vi "Header.vi"() -> ()   [LabVIEW 2011]
uses:
  <vilib>/Utility/miscctls.llb/LVPointTypeDef.ctl
  Globals/Global VI.vi
  Globals/Global Recipe.vi
panel:
  out "System Status :":u16(ring) items=["NOT READY", "E-STOPPED", "FAULTED", "PAUSING...", "PAUSED", "IDLE", "RUNNING", "UNCALIBRATED", "CALIBRATING...", "POWER OFF", "POWERING ON...", "MANUAL MODE", "CONNECTING..."]
  out "Faulted":bool
  in  "Previous Button":bool
  in  "Next Button":bool
  in  "Last Button":bool
  in  "First Button":bool
  in  "Login Button":bool
  out "Date/Time":string="Date\nTime"
  out "String":string
  out "Operator":string
  out "System Info":string="System Idle"
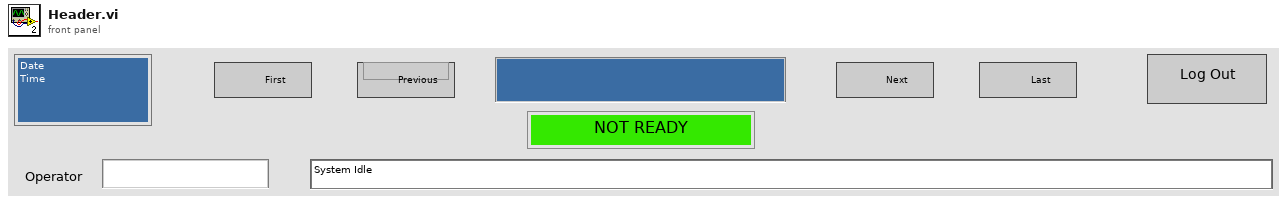
[diagram p1: front panel]
types:
  T1 = typedef "LVPointTypeDef.ctl" = cluster{"Horizontal":i16, "Vertical":i16}
  T2 = enum16{"Always On", "Always Off", "Off While Running"}
  T3 = typedef "LVRectTypeDef.ctl" = cluster{"left":i16, "top":i16, "right":i16, "bottom":i16}
  T4 = typedef "LVAllMonitorsDisplayTypeDef.ctl" = cluster{"Bounds":cluster{"Left":i16, "Top":i16, "Right":i16, "Bottom":i16}, "Depth":i16}[]
  T5 = cluster{"Bounds":cluster{"Left":i16, "Top":i16, "Right":i16, "Bottom":i16}, "Depth":i16}
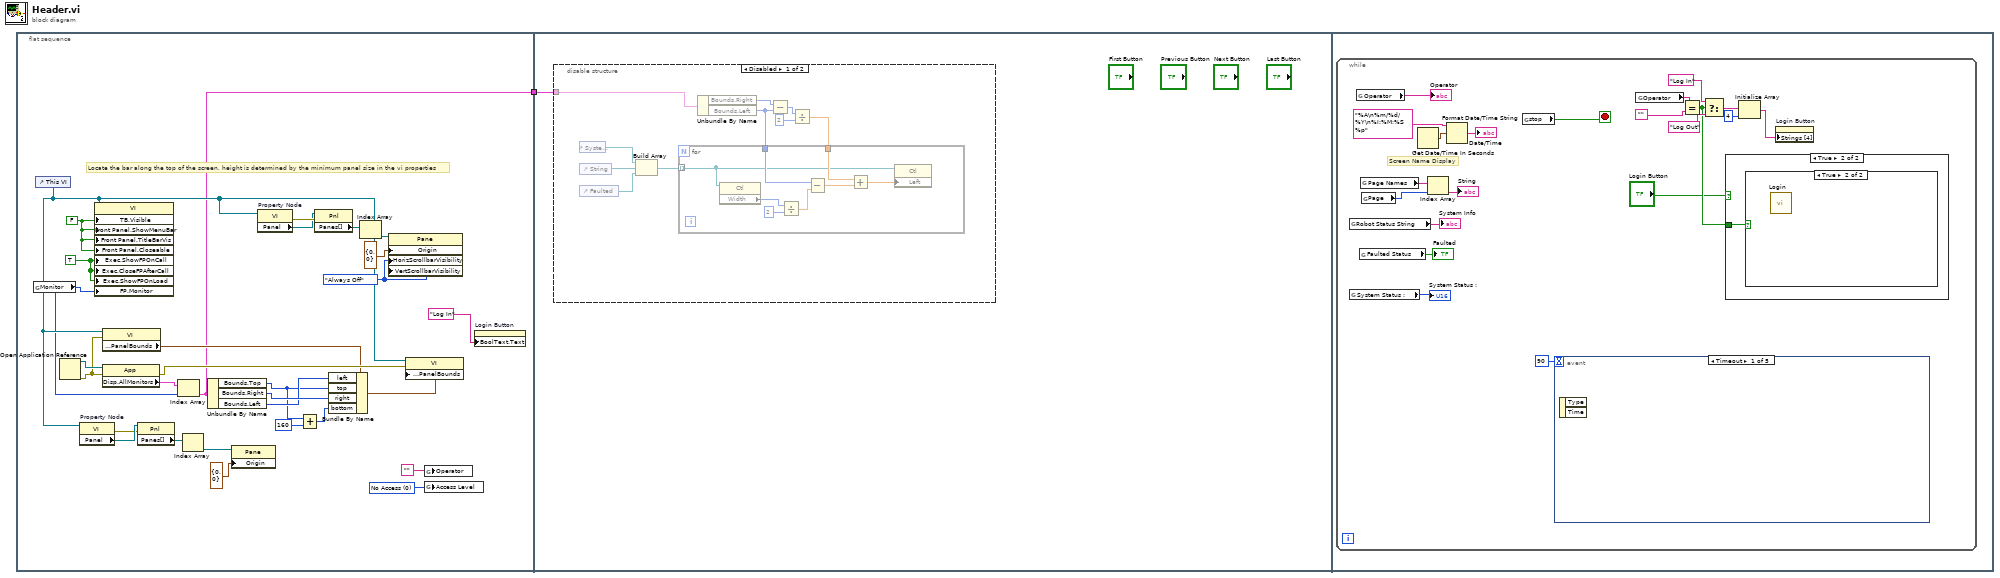
[diagram p0: block diagram]
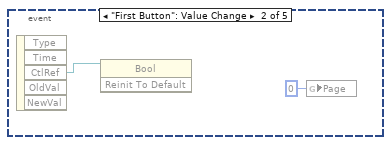
[diagram p3: hidden frame]
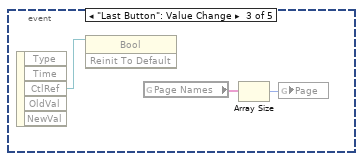
[diagram p4: hidden frame]
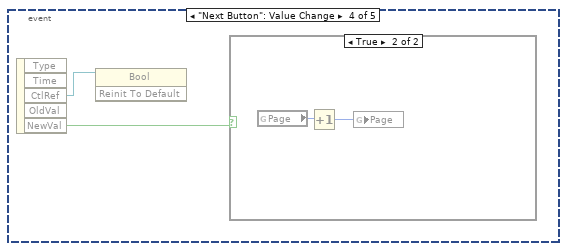
[diagram p5: hidden frame]
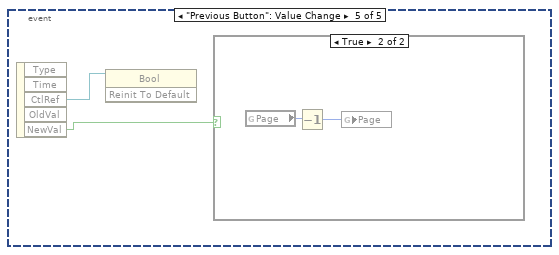
[diagram p7: hidden frame]
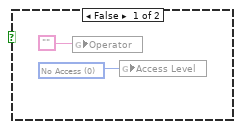
[diagram p10: hidden frame]
diagram:
  n1 = flat-sequence {
    tunnel: [w3] -> w1
    tunnel: w1 -> [w32]
    frame #0 {
      w6 = u16 0 items=["No Access", "Operator", "Engineer/Tech"] ("Access Level")
      w9 = TRUE ("Execution:Show Front Panel On Call")
      w8 = FALSE ("Tool Bar:Visible")
      w11 = T2."Always Off" ("Horizontal Scrollbar Visibility")
      # "Locate the bar along the top of the screen, height is determined by the minimum panel size in the vi properties"
      n2 = global read "Global VI.vi" "Monitor"() -> (w2:u16)
      n3 = control-ref of="This VI"() -> (w7:refnum<vi>)
      n4 = Open Application Reference() -> (0:w27:errorcluster, 3:w28:refnum<vi>)  [unwired: 4 in]
      n5 = property on="Property Node" class="VI"(reference=w7) -> (error out=w25:errorcluster, "Panel"=w26:refnum<vi>)  [unwired: 1 in, 1 out]
      n6 = property class="VI"(reference=w7, "TB.Visible"=w8, "Front Panel.ShowMenuBar"=w8, "Front Panel.TitleBarVis"=w8, "Front Panel.Closeable"=w8, "Exec.ShowFPOnCall"=w9, "Exec.CloseFPAfterCall"=w9, "Exec.ShowFPOnLoad"=w9, "FP.Monitor"=w2) -> ()  [unwired: 1 in, 2 out]
      n7 = property class="VI"(reference=w7, error in=w27) -> ("Front Panel.PanelBounds"=w21:T3)  [unwired: 2 out]
      n8 = property class="App"(reference=w28, error in=w27) -> (error out=w30:errorcluster, "Disp.AllMonitors"=w31:T4)  [unwired: 1 out]
      n9 = property class="Pnl"(reference=w26, error in=w25) -> ("Panes[]"=w24:refnum<vi>[])  [unwired: 2 out]
      n10 = Index Array(array=w31, index=w2) -> (element=w3:T5)
      n11 = Index Array "Index Array"(array=w24) -> (element=w23:refnum<vi>)  [unwired: 1 in]
      n12 = Unbundle By Name(w3) -> ("Bounds.Top"=w18:i16, "Bounds.Right"=w20:i16, "Bounds.Left"=w19:i16)
      n13 = property class="Pane"(reference=w23, "Origin"=T1 {"Horizontal"=0, "Vertical"=0}) -> ()  [unwired: 1 in, 2 out]
      n14 = property on="Property Node" class="VI"(reference=w7) -> (error out=w13:errorcluster, "Panel"=w12:refnum<vi>)  [unwired: 1 in, 1 out]
      n15 = Add(x=w18, y=i16 160) -> (x+y=w16:i16)
      n16 = property class="Pnl"(reference=w12, error in=w13) -> ("Panes[]"=w14:refnum<vi>[])  [unwired: 2 out]
      n17 = Bundle By Name(cluster=w21, "left"=w19, "top"=w18, "right"=w20, "bottom"=w16) -> (w29:T3)
      n18 = Index Array "Index Array"(array=w14) -> (element=w15:refnum<vi>)  [unwired: 1 in]
      n19 = property class="Pane"(reference=w15, "Origin"=T1 {"Horizontal"=0, "Vertical"=0}, "HorizScrollbarVisibility"=w11, "VertScrollbarVisibility"=w11) -> ()  [unwired: 1 in, 2 out]
      n20 = property on="Property Node" class="VI"(reference=w7, error in=w30, "Front Panel.PanelBounds"=w29) -> ()  [unwired: 2 out]
      n21 = global write "Global VI.vi" "Operator"("") -> ()
      n22 = global write "Global VI.vi" "Access Level"(w6) -> ()
      n23 = property on="Login Button" class="Bool"("BoolText.Text"="Log In" ("Boolean Text.Text")) -> ()  [unwired: 2 in, 2 out]
    }
    frame #1 {
      n24 = disable-structure shown="Disabled" {
        disable-tunnel: w32 -> [w39 _]
        frame Disabled {
          n25 = control-ref of="System Status :"() -> (w36:refnum<vi>)
          n26 = control-ref of="String"() -> (w35:refnum<vi>)
          n27 = control-ref of="Faulted"() -> (w34:refnum<vi>)
          n28 = Build Array(w36, w35, w34) -> (w33:refnum<vi>[])
          n29 = Unbundle By Name(w39) -> ("Bounds.Right"=w40:i16, "Bounds.Left"=w37:i16)
          n30 = Subtract(x=w40, y=w37) -> (x-y=w42:i16)
          n31 = Divide(x=w42, y=u32 2) -> (x/y=w38:dbl)
          n32 = for {
            tunnel: w38 -> [w45]
            tunnel: w37 -> [w44]
            tunnel: w33 -> [w43] mode=indexing
            n33 = property class="Ctl"(reference=w43) -> ("Width"=w49:u32)  [unwired: 1 in, 2 out]
            n34 = Divide(x=w49, y=u32 2) -> (x/y=w48:dbl)
            n35 = Subtract(x=w44, y=w48) -> (x-y=w47:dbl)
            n36 = Add(x=w45, y=w47) -> (x+y=w46:dbl)
            n37 = property class="Ctl"(reference=w43, "Left"=w46) -> ()  [unwired: 1 in, 2 out]
          }
        }
        frame Enabled {
        }
      }
    }
    frame #2 {
      n38 = while {
        stop <- w62 stop-if-true
        # "Screen Name Display"
        n39 = global read "Global VI.vi" "Robot Status String"() -> (→"System Info":string)
        n40 = global read "Global Recipe.vi" "System Status :"() -> (→"System Status :":u16)
        n41 = global read "Global VI.vi" "Operator"() -> (→"Operator":string)
        n42 = global read "Global VI.vi" "Faulted Status"() -> (→"Faulted":bool)
        n43 = global read "Global VI.vi" "Page Names"() -> (w68:string[])
        n44 = global read "Global VI.vi" "Page"() -> (w67:i16)
        n45 = Get Date/Time In Seconds() -> (seconds since 1Jan1904=w71:timestamp)
        n46 = Index Array(array=w68, index=w67) -> (element=→"String":string)
        n47 = Format Date/Time String(time format string (%c)="%A\n%m/%d/%Y\n%I:%M:%S %p" ("HMI Date Format String"), seconds (now)=w71) -> (date/time string=→"Date/Time":string)  [unwired: 1 in]
        n48 = global read "Global VI.vi" "stop"() -> (w62:bool)
        n49 = event shown="[0] Timeout" {
          selector: _ -> [_ _ _ _ _]
          dyn-events: _ -> [_ _ _ _ _]
          timeout: 90 -> [_ _ _ _ _]
          event Timeout {
            n50 = event-data() -> ()  [unwired: 1 in, 2 out]
          }
          event "First Button": Value Change {
            n51 = event-data() -> ("CtlRef"=w72:refnum<vi>)  [unwired: 1 in, 4 out]
            n52 = invoke class="Bool" method="Reinit To Default"(reference=w72) -> ()  [unwired: 2 in, 3 out]
            n53 = global write "Global VI.vi" "Page"(i16 0 ("Page")) -> ()
          }
          event "Last Button": Value Change {
            n54 = event-data() -> ("CtlRef"=w74:refnum<vi>)  [unwired: 1 in, 4 out]
            n55 = invoke class="Bool" method="Reinit To Default"(reference=w74) -> ()  [unwired: 2 in, 3 out]
            n56 = global read "Global VI.vi" "Page Names"() -> (w75:string[])
            n57 = Array Size(array=w75) -> (size(s)=w76:i32)
            n58 = global write "Global VI.vi" "Page"(w76) -> ()
          }
          event "Next Button": Value Change {
            n59 = event-data() -> ("CtlRef"=w77:refnum<vi>, "NewVal"=w78:bool)  [unwired: 1 in, 3 out]
            n60 = invoke class="Bool" method="Reinit To Default"(reference=w77) -> ()  [unwired: 2 in, 3 out]
            n61 = case shown="True" w78 {
              frame False {
              }
              frame True {
                n62 = global read "Global VI.vi" "Page"() -> (w80:i16)
                n63 = Increment(x=w80) -> (x+1=w79:i16)
                n64 = global write "Global VI.vi" "Page"(w79) -> ()
              }
            }
          }
          event "Previous Button": Value Change {
            n65 = event-data() -> ("CtlRef"=w81:refnum<vi>, "NewVal"=w82:bool)  [unwired: 1 in, 3 out]
            n66 = invoke class="Bool" method="Reinit To Default"(reference=w81) -> ()  [unwired: 2 in, 3 out]
            n67 = case shown="True" w82 {
              frame False {
              }
              frame True {
                n68 = global read "Global VI.vi" "Page"() -> (w84:i16)
                n69 = Decrement(x=w84) -> (x-1=w83:i16)
                n70 = global write "Global VI.vi" "Page"(w83) -> ()
              }
            }
          }
        }
        n71 = global read "Global VI.vi" "Operator"() -> (w60:string)
        n72 = Equal?(x=w60, y="") -> (x = y?=w55:bool)
        n73 = Select(t="Log In" ("Robot Status String"), s=w55, f="Log Out") -> (s? t:f=w58:string)
        n74 = case shown="True" "Login Button" {
          tunnel: w55 -> [_ w85]
          frame False {
          }
          frame True {
            n75 = case shown="True" w85 {
              frame False {
                w86 = u16 0 items=["No Access", "Operator", "Engineer/Tech"] ("Access Level")
                n76 = global write "Global VI.vi" "Operator"("") -> ()
                n77 = global write "Global VI.vi" "Access Level"(w86) -> ()
              }
              frame True {
                n78 = call "Login.vi"() -> ()  [unwired: 12 in]
              }
            }
          }
        }
        n79 = Initialize Array(w58, 4 ("dimension size")) -> (w54:string[])
        n80 = property on="Login Button" class="Bool"("Strings [4]"=w54) -> ()  [unwired: 2 in, 2 out]
      }
    }
  }
